vi "Close Report.vi"(2 "error in (no error)":errorcluster, 3 "Save Changes?":bool, 4 "Report Ref In":T1) -> (0 "error out":errorcluster, 1 "Report Ref Out":T1)   [LabVIEW 2026, in "XCel Report Engine.lvlib"]
uses:
  XCel Report Engine.lvlib
  Controls/Report Ref.ctl
  C:/Users/m.santucci/Documents/ChatGPT/LV_REPORT_ENGINE/.net/src/XCelReportEngine/bin/Release/net48/XCelReportEngine.dll
  .net/src/XCelReportEngine/bin/Release/net48/XCelReportEngine.dll
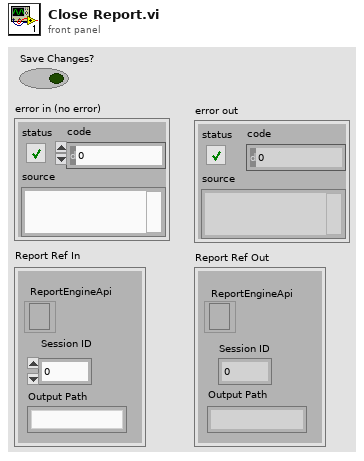
[diagram p1: front panel]
types:
  T1 = typedef "XCel Report Engine.lvlib/Report Ref.ctl" = cluster{"Session ID":i32, "Output Path":string, "ReportEngineApi":refnum<k24>}
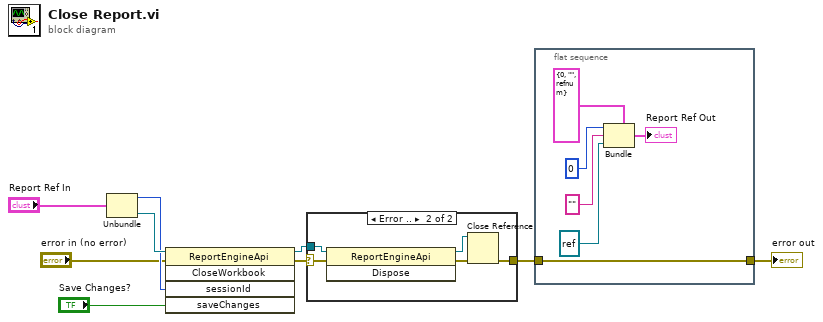
[diagram p0: block diagram]
diagram:
  n1 = Unbundle("Report Ref In") -> ("Session ID"=w7:i32, "ReportEngineApi"=w8:refnum<k24>)  [unwired: 1 out]
  n2 = invoke class="ReportEngineApi" method="CloseWorkbook"(reference=w8, error in="error in (no error)", "sessionId"=w7, "saveChanges"="Save Changes?") -> (reference out=w3:refnum<k24>, error out=w4:errorcluster)  [unwired: 1 in, 3 out]
  n3 = case shown="Error .." w4 {
    selector: w4 -> [w10 w13]
    tunnel: w3 -> [_ w15]
    tunnel: [w10 w11] -> w2
    frame No Error {
    }
    frame Error {
      n4 = invoke class="ReportEngineApi" method="Dispose"(reference=w15, error in=w13) -> (reference out=w14:refnum<k24>, error out=w12:errorcluster)  [unwired: 1 in, 1 out]
      n5 = Close Reference(reference=w14, error in (no error)=w12) -> (error out=w11:errorcluster)
    }
  }
  n6 = flat-sequence {
    tunnel: w2 -> [w21]
    tunnel: [w21] -> w1
    frame #0 {
      n7 = Bundle(cluster=T1 {"Session ID"=0, "Output Path"="", "ReportEngineApi"=refnum} ("Report Ref"), "Session ID"=0, "Output Path"="", "ReportEngineApi"=refnum<k24> refnum) -> (→"Report Ref Out":T1)
    }
  }
  "error out" <- w1
